vi "Create and Read AI.vi"(8 "error in":errorcluster, 10 "initial channel settings":T1[](array[typedef]), 11 "module test in":refnum<class "Module Test.lvclass">) -> (0 "error out":errorcluster, 2 "read channel settings":T1[](array[typedef]), 3 "module test out":refnum<class "Module Test.lvclass">)   [LabVIEW 2019, in "Module Test.lvclass"]
uses:
  Module Test.lvclass
  Scripting/Modules/Mode Classes/Controls/analog channel settings.ctl
  Scripting/Scan Engine Scripting.lvlib
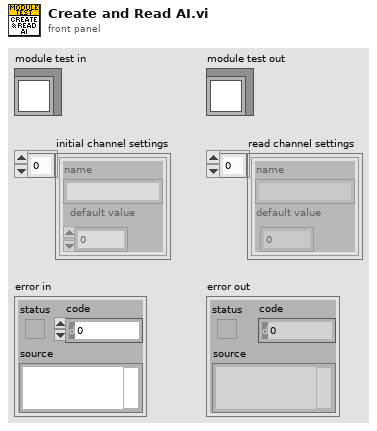
[diagram p1: front panel]
types:
  T1 = typedef "Scan Engine Scripting.lvlib/analog channel settings.ctl" = cluster{"name":string, "default value":dbl}
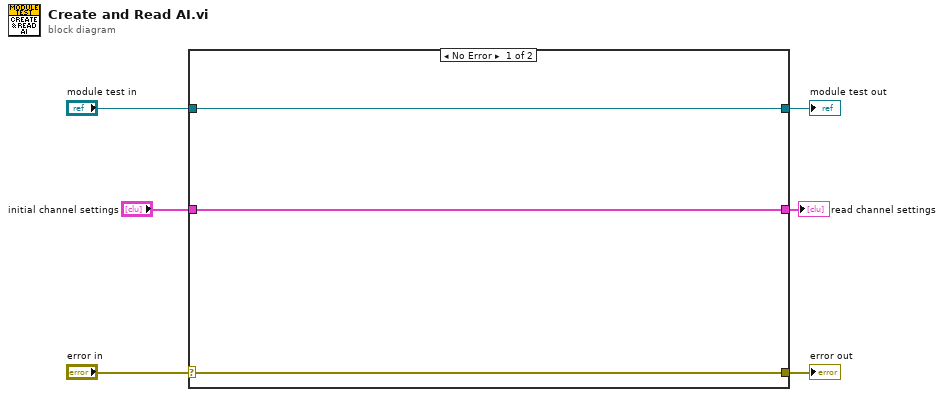
[diagram p0: block diagram]
diagram:
  n1 = case shown="No Error" "error in" {
    selector: "error in" -> [w8 w12]
    tunnel: [w8 w12] -> w5
    tunnel: [w9 w11] -> w3
    tunnel: "module test in" -> [w9 w11]
    tunnel: "initial channel settings" -> [w7 w10]
    tunnel: [w7 w10] -> w1
    frame No Error {
    }
    frame Error {
    }
  }
  "error out" <- w5
  "module test out" <- w3
  "read channel settings" <- w1
